vi "saveImage.vi"(6 "bit depth":enum16{"16bits", "14bits", "12bits", "8bits"}(ring), 7 "session in":refnum<k35>, 8 "reff ROI":i32[](array[numeric]), 9 "main ROI":i32[](array[numeric]), 10 "appended path":string, 11 "Refnum in":T1) -> (0 "error out":errorcluster, 5 "session out":refnum<k35>)   [LabVIEW 2023]
uses:
  <vilib>/vision/Image Controls.llb/IMAQ Image.ctl
panel:
  out "numpy filename":string
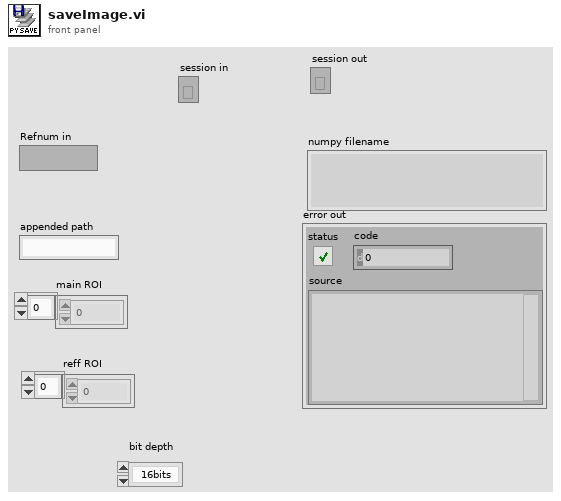
[diagram p1: front panel]
types:
  T1 = typedef "IMAQ Image.ctl" = refnum<image>
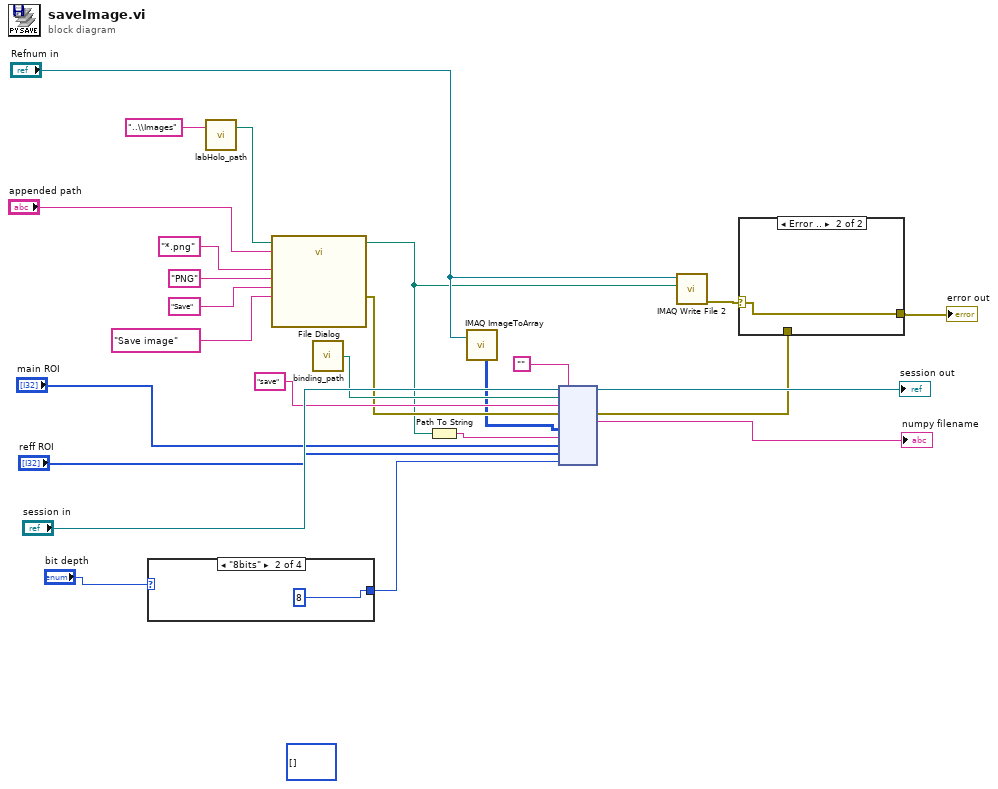
[diagram p0: block diagram]
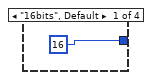
[diagram p3: hidden frame]
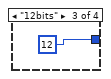
[diagram p4: hidden frame]
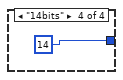
[diagram p5: hidden frame]
diagram:
  (unwired) u16[][] [] ("image")
  n1 = case shown="\"8bits\"" "bit depth" {
    tunnel: [16 8 12 14] -> w4
    frame "16bits", Default {
    }
    frame "8bits" {
    }
    frame "12bits" {
    }
    frame "14bits" {
    }
  }
  n2 = call "labHolo_path.vi"("sub folder or file (str)"="..\\Images") -> ("labHolo path"=w24:path)  [unwired: 1 in, 1 out]
  n3 = call "File Dialog"("start path"=w24, "prompt"="Save image", "button label"="Save", "default name"="appended path", "pattern (all files)"="*.png", "pattern label"="PNG") -> ("selected path"=w12:path, "error out"=w15:errorcluster)  [unwired: 6 in, 2 out]
  n4 = call "binding_path.vi"() -> ("appended path"=w17:path)
  n5 = Path To String(path=w12) -> (string=w11:string)
  n6 = call "IMAQ ImageToArray"("Image"="Refnum in") -> ("Image Pixels (U16)"=w13:u16[][])  [unwired: 3 in, 4 out]
  n7 = node("session in", w17, "save" ("function name"), w15, "", w13, w11, "main ROI", "reff ROI", w4) -> (→"session out":refnum<k35>, w2:errorcluster, →"numpy filename":string)  [unwired: 5 in, 2 out]
  n8 = call-poly "IMAQ Write File 2"("File Path"=w12, "Image"="Refnum in") -> ("error out"=w3:errorcluster)  [unwired: 8 in, 1 out]
  n9 = case shown="Error .." w3 {
    selector: w3 -> [_ w31]
    tunnel: [w30 w31] -> w1
    tunnel: w2 -> [w30 _]
    frame No Error {
    }
    frame Error {
    }
  }
  "error out" <- w1
